vi "get_list_of_configurations.vi"(8 "error in (no error)":errorcluster, 11 "GenericComponent in":refnum<class "GenericComponent.lvclass">) -> (0 "error out":errorcluster, 2 "configurations":string[](array[string]), 3 "GenericComponent out":refnum<class "GenericComponent.lvclass">)   [LabVIEW 2010, in "GenericComponent.lvclass"]
uses:
  GenericComponent.lvclass
  <vilib>/regexp/Match Regular Expression.xnode
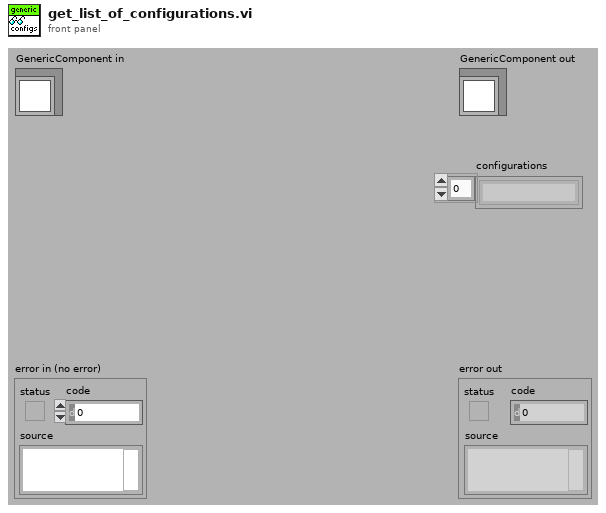
[diagram p1: front panel]
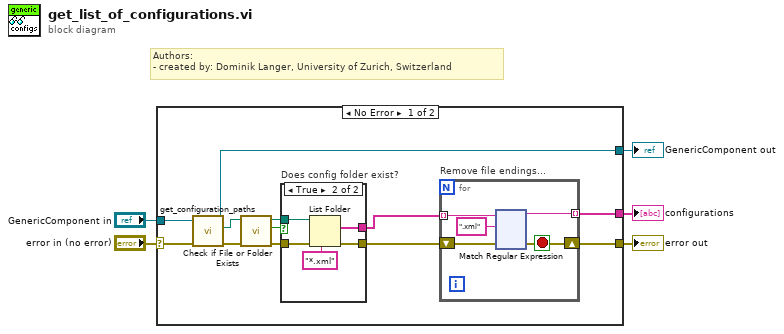
[diagram p0: block diagram]
diagram:
  # "Authors: \n- created by: Dominik Langer, University of Zurich, Switzerland"
  n1 = case shown="No Error" "error in (no error)" {
    selector: "error in (no error)" -> [w17 w141]
    tunnel: [w8 w141] -> w4
    tunnel: [w15 w140] -> w2
    tunnel: "GenericComponent in" -> [w16 w140]
    tunnel: [w6 _] -> w1
    frame No Error {
      n2 = call-dynamic "get_configuration_paths.vi"("error in (no error)"=w17, "GenericComponent in"=w16) -> ("error out"=w13:errorcluster, "configuration directory for a specific component"=w14:path, "GenericComponent out"=w15:refnum<class "GenericComponent.lvclass">)  [unwired: 2 in, 5 out]
      n3 = call <vilib>:"Check if File or Folder Exists.vi"("error in (no error)"=w13, "path"=w14) -> ("error out"=w12:errorcluster, "file or folder exists?"=w10:bool, "dup path"=w11:path)  [unwired: 7 out]
      n4 = case "Does config folder exist?" shown="True" w10 {
        tunnel: w12 -> [w134 w139]
        tunnel: [w134 w138] -> w9
        tunnel: w11 -> [_ w137]
        tunnel: [_ w136] -> w7
        frame False {
        }
        frame True {
          n5 = List Folder(path=w137, pattern="*.xml", error in=w139) -> (filenames=w136:string[], error out=w138:errorcluster)  [unwired: 3 out]
        }
      }
      n6 = for "Remove file endings..." {
        shift-right: [w21] -> w8
        shift-left: w9 -> [w22]
        tunnel: w7 -> [w20] mode=indexing
        tunnel: [w19] -> w6 mode=indexing
        stop <- w21 stop-if-true
        n7 = xnode "Match Regular Expression"("input string"=w20, "regular expression"=".xml", "error in"=w22) -> ("before match"=w19:string, "error out"=w21:errorcluster)  [unwired: 3 in, 3 out]
      }
    }
    frame Error {
    }
  }
  "error out" <- w4
  "GenericComponent out" <- w2
  "configurations" <- w1
